vi "Initialize-processing-and-black-buffer-refs.vi"(8 "error in (no error)":errorcluster, 9 "Number of cameras":i32, 10 "Image buffer size":i32, 11 "Buffers in":refnum<class "CV-Buffers.lvclass">) -> (0 "error out":errorcluster, 3 "Buffers out":refnum<class "CV-Buffers.lvclass">)   [LabVIEW 2013, in "CameraVision.lvlib" / "CV-Buffers.lvclass"]
uses:
  CV-Buffers.lvclass
  CV-Buffers.lvclass/CV-Buffers.ctl
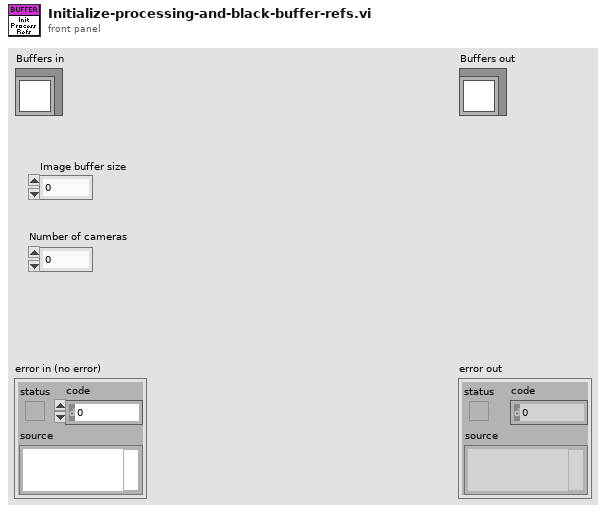
[diagram p1: front panel]
types:
  T1 = typedef "Image Type" = u32
  T2 = typedef "IMAQ Image.ctl" = refnum<image>
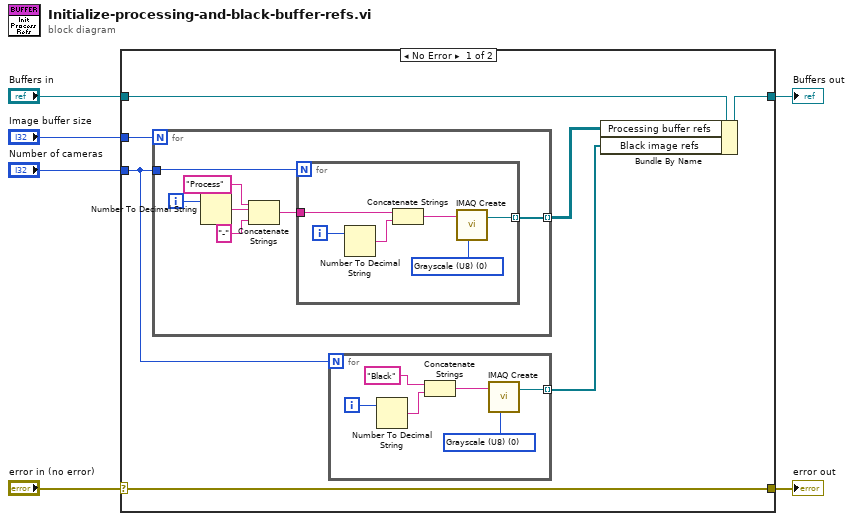
[diagram p0: block diagram]
diagram:
  n1 = case shown="No Error" "error in (no error)" {
    selector: "error in (no error)" -> [w12 w34]
    tunnel: [w12 w34] -> w5
    tunnel: [w11 w33] -> w3
    tunnel: "Buffers in" -> [w13 w33]
    tunnel: "Image buffer size" -> [w9 _]
    tunnel: "Number of cameras" -> [w8 _]
    frame No Error {
      n2 = for {
        N: w9 -> [_]
        tunnel: [w21] -> w10 mode=indexing
        tunnel: w8 -> [w20]
        i -> [w26]
        n3 = Number To Decimal String(number=w26) -> (decimal integer string=w25:string)  [unwired: 1 in]
        n4 = Concatenate Strings("Process" ("string"), w25, "-" ("string")) -> (w22:string)
        n5 = for {
          N: w20 -> [_]
          tunnel: w22 -> [w30]
          tunnel: [w27] -> w21 mode=indexing
          i -> [w32]
          w29 = T1 0 items=["Grayscale (U8)", "Grayscale (I16)", "Grayscale (SGL)", "Complex (CSG)", "RGB (U32)", "HSL (U32)", "RGB (U64)", "Grayscale (U16)"] ("Image Type")
          n6 = Number To Decimal String(number=w32) -> (decimal integer string=w31:string)  [unwired: 1 in]
          n7 = Concatenate Strings(w30, w31) -> (w28:string)
          n8 = call "IMAQ Create"("Image Name"=w28, "Image Type"=w29) -> ("New Image"=w27:T2)  [unwired: 3 in, 1 out]
        }
      }
      n9 = for {
        N: w8 -> [_]
        tunnel: [w15] -> w7 mode=indexing
        i -> [w19]
        w17 = T1 0 items=["Grayscale (U8)", "Grayscale (I16)", "Grayscale (SGL)", "Complex (CSG)", "RGB (U32)", "HSL (U32)", "RGB (U64)", "Grayscale (U16)"] ("Image Type")
        n10 = Number To Decimal String(number=w19) -> (decimal integer string=w18:string)  [unwired: 1 in]
        n11 = Concatenate Strings("Black" ("string"), w18) -> (w16:string)
        n12 = call "IMAQ Create"("Image Name"=w16, "Image Type"=w17) -> ("New Image"=w15:T2)  [unwired: 3 in, 1 out]
      }
      n13 = Bundle By Name(cluster=w13, "Processing buffer refs"=w10, "Black image refs"=w7) -> (w11:refnum<class "CV-Buffers.lvclass">)
    }
    frame Error {
    }
  }
  "error out" <- w5
  "Buffers out" <- w3
